vi "create_file_name (SubVI).vi"(0 "Dipole average settings":T1, 1 "stage on?":bool, 2 "file_idx":i32, 4 "QWP":bool, 5 "num files per step":i32, 6 "num files":i32, 7 "base name":string, 8 "Path":path, 9 "Process List":T2) -> (3 "out path":path)   [LabVIEW 2016]
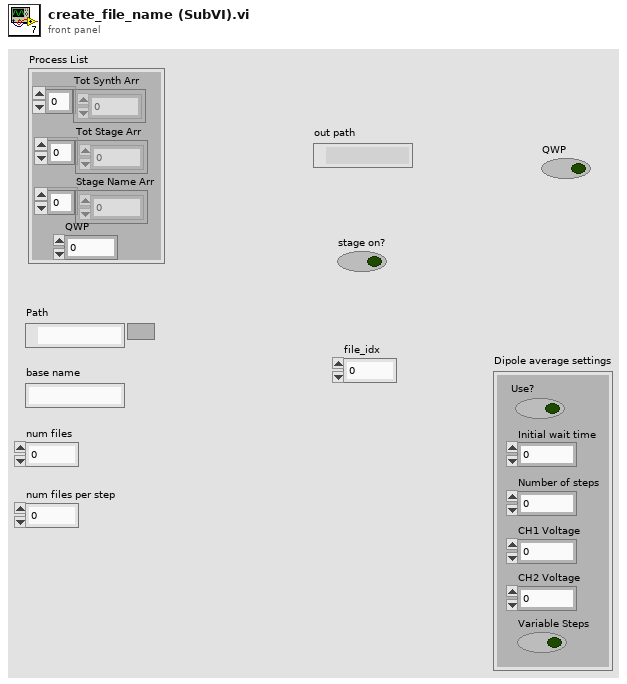
[diagram p1: front panel]
types:
  T1 = cluster{"Initial wait time":dbl, "Number of steps":i32, "CH1 Voltage":dbl, "Use?":bool, "CH2 Voltage":dbl, "Variable Steps":bool}
  T2 = cluster{"Tot Synth Arr":dbl[], "Tot Stage Arr":dbl[], "Stage Name Arr":dbl[], "QWP":dbl}
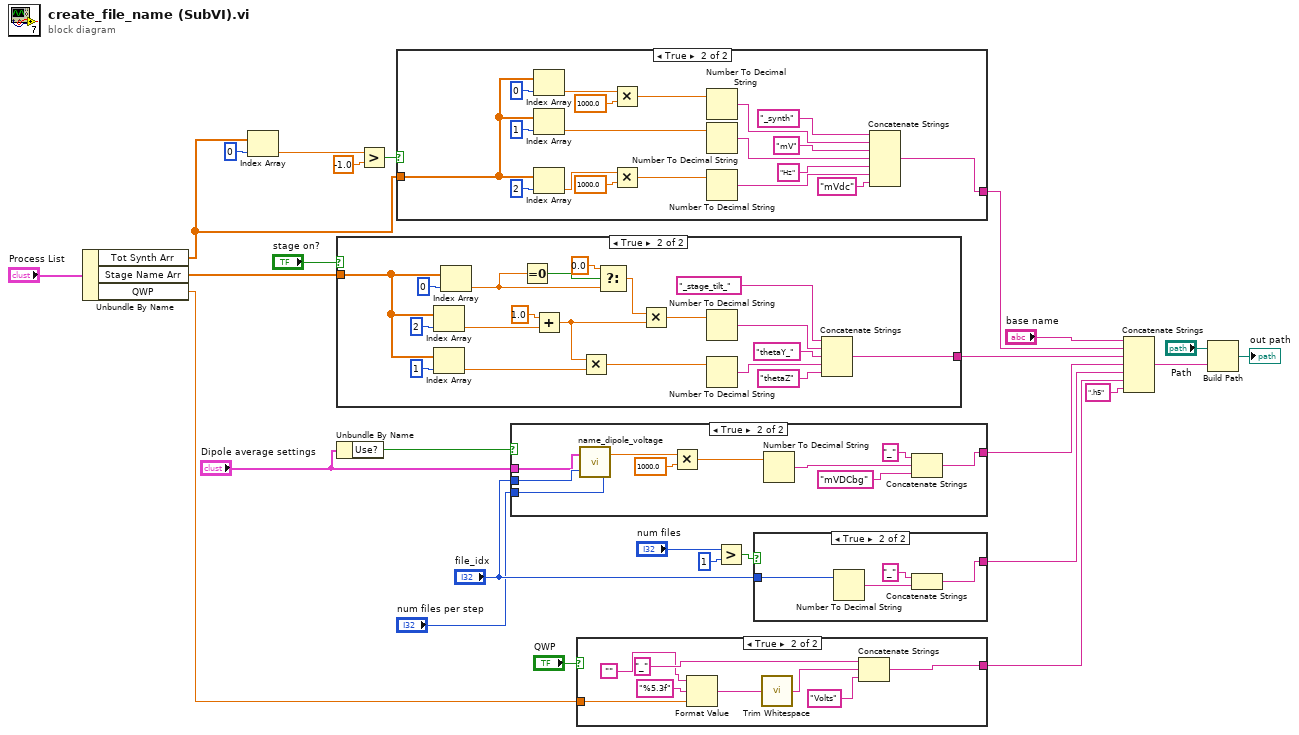
[diagram p0: block diagram]
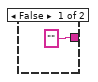
[diagram p2: hidden frame]
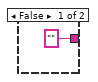
[diagram p3: hidden frame]
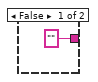
[diagram p4: hidden frame]
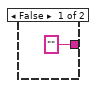
[diagram p5: hidden frame]
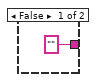
[diagram p6: hidden frame]
diagram:
  n1 = Unbundle By Name("Process List") -> ("Tot Synth Arr"=w22:dbl[], "Stage Name Arr"=w13:dbl[], "QWP"=w4:dbl)
  n2 = Index Array(array=w22, index=0) -> (element=w24:dbl)
  n3 = case shown="True" "stage on?" {
    tunnel: w13 -> [_ w39]
    tunnel: ["" w41] -> w14
    frame False {
    }
    frame True {
      n4 = Index Array(array=w39, index=2) -> (element=w35:dbl)
      n5 = Index Array(array=w39, index=1) -> (element=w36:dbl)
      n6 = Index Array(array=w39, index=0) -> (element=w29:dbl)
      n7 = Equal To 0?(x=w29) -> (x = 0?=w30:bool)
      n8 = Add(x=1.0, y=w35) -> (x+y=w33:dbl)
      n9 = Multiply(x=w33, y=w36) -> (x*y=w37:dbl)
      n10 = Select(t=0.0 ("f"), s=w30, f=w29) -> (s? t:f=w31:dbl)
      n11 = Multiply(x=w31, y=w33) -> (x*y=w38:dbl)
      n12 = Number To Decimal String(number=w38) -> (decimal integer string=w45:string)  [unwired: 1 in]
      n13 = Number To Decimal String(number=w37) -> (decimal integer string=w43:string)  [unwired: 1 in]
      n14 = Concatenate Strings("_stage_tilt_", w45, "thetaY_" ("string"), w43, "thetaZ" ("string")) -> (w41:string)
    }
  }
  n15 = Unbundle By Name("Dipole average settings") -> ("Use?"=w8:bool)
  n16 = Greater?(x=w24, y=-1.0) -> (0:w23:bool)
  n17 = case shown="True" w23 {
    tunnel: w22 -> [_ w68]
    tunnel: ["" w50] -> w20
    frame False {
    }
    frame True {
      n18 = Index Array(array=w68, index=0) -> (element=w63:dbl)
      n19 = Index Array(array=w68, index=1) -> (element=w64:dbl)
      n20 = Index Array(array=w68, index=2) -> (element=w59:dbl)
      n21 = Multiply(x=w63, y=1000.0) -> (x*y=w62:dbl)
      n22 = Multiply(x=w59, y=1000.0) -> (x*y=w58:dbl)
      n23 = Number To Decimal String(number=w62) -> (decimal integer string=w56:string)  [unwired: 1 in]
      n24 = Number To Decimal String(number=w64) -> (decimal integer string=w54:string)  [unwired: 1 in]
      n25 = Number To Decimal String(number=w58) -> (decimal integer string=w52:string)  [unwired: 1 in]
      n26 = Concatenate Strings("_synth" ("string"), w56, "mV" ("string"), w54, "Hz" ("string"), w52, "mVdc" ("string")) -> (w50:string)
    }
  }
  n27 = case shown="True" w8 {
    tunnel: "file_idx" -> [_ w79]
    tunnel: "Dipole average settings" -> [_ w78]
    tunnel: ["" w74] -> w9
    tunnel: "num files per step" -> [_ w73]
    frame False {
    }
    frame True {
      n28 = call "name_dipole_voltage.vi"("Num files"=w73, "iteration number"=w79, "Dipole average settings"=w78) -> ("Voltage name"=w72:dbl)
      n29 = Multiply(x=w72, y=1000.0) -> (x*y=w70:dbl)
      n30 = Number To Decimal String(number=w70) -> (decimal integer string=w77:string)  [unwired: 1 in]
      n31 = Concatenate Strings("_" ("string"), w77, "mVDCbg" ("string")) -> (w74:string)
    }
  }
  n32 = case shown="True" "QWP" {
    tunnel: w4 -> [_ w86]
    tunnel: ["" w88] -> w2
    frame False {
    }
    frame True {
      n33 = Format Value(string ("")="", format string="%5.3f", value (0)=w86) -> (output string=w85:string)
      n34 = call <vilib>:"Trim Whitespace.vi"("string"=w85) -> ("trimmed string"=w83:string)  [unwired: 1 in]
      n35 = Concatenate Strings("_" ("string"), w83, "Volts" ("string")) -> (w88:string)
    }
  }
  n36 = Greater?(x="num files", y=1) -> (0:w15:bool)
  n37 = case shown="True" w15 {
    tunnel: "file_idx" -> [_ w92]
    tunnel: ["" w90] -> w10
    frame False {
    }
    frame True {
      n38 = Number To Decimal String(number=w92) -> (decimal integer string=w91:string)  [unwired: 1 in]
      n39 = Concatenate Strings("_" ("string"), w91) -> (w90:string)
    }
  }
  n40 = Concatenate Strings("base name", w20, w14, w9, w10, w2, ".h5" ("string")) -> (w19:string)
  n41 = Build Path(base path="Path", name or relative path=w19) -> (appended path=→"out path":path)
